vi "Write Display settings.vi"(8 "error in (no error)":errorcluster, 10 "Display settings":T1={"Min. Thresh."=0.0, "X"=0.0, "Y"=0.0, "ShowLineout"=FALSE, "ScaleParts"=10, "ShowLegende"=FALSE, "Target Cross"=FALSE, "Centroid Cross"=FALSE, "Target color"=16777226, "Centroid color"=16711680, "calibr. µm/px"=0.0}, 11 "Display Settings Dialog in":refnum<class "Display Settings Dialog.lvclass">) -> (0 "error out":errorcluster, 3 "Display Settings Dialog out":refnum<class "Display Settings Dialog.lvclass">)   [LabVIEW 2014, in "Display Settings Dialog.lvlib" / "Display Settings Dialog.lvclass"]
uses:
  Display Settings Dialog.lvclass
  HIJ Vision Display/HIJ Vision Display/DisplaySettings.ctl
  Display Settings Dialog.lvclass/Display Settings Dialog.ctl
  HIJ Vision Display/HIJ Vision Display/HIJ Vision Display.lvclass
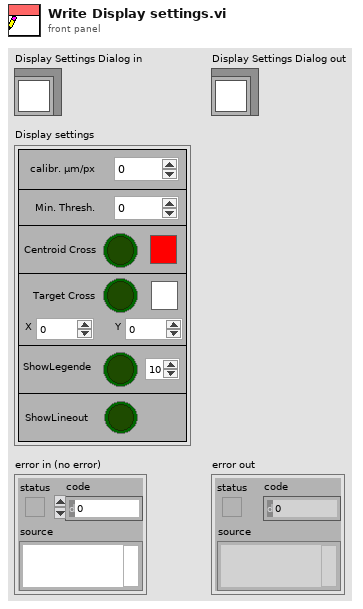
[diagram p1: front panel]
types:
  T1 = typedef "HIJ Vision Display.lvlib/HIJ Vision Display.lvclass/DisplaySettings.ctl" = cluster{"Min. Thresh.":sgl, "X":dbl, "Y":dbl, "ShowLineout":bool, "ScaleParts":i32, "ShowLegende":bool, "Target Cross":bool, "Centroid Cross":bool, "Target color":u32, "Centroid color":u32, "calibr. µm/px":sgl[unit]}
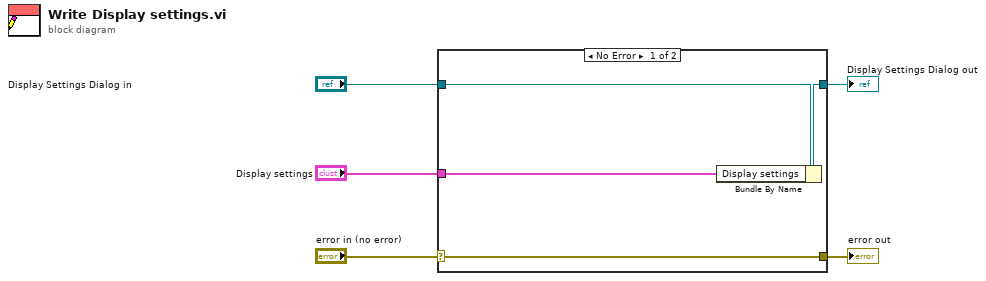
[diagram p0: block diagram]
diagram:
  n1 = case shown="No Error" "error in (no error)" {
    selector: "error in (no error)" -> [w9 w10]
    tunnel: [w9 w10] -> w4
    tunnel: [w7 w11] -> w2
    tunnel: "Display Settings Dialog in" -> [w8 w11]
    tunnel: "Display settings" -> [w6 _]
    frame No Error {
      n2 = Bundle By Name(cluster=w8, "Display settings"=w6) -> (w7:refnum<class "Display Settings Dialog.lvclass">)
    }
    frame Error {
    }
  }
  "error out" <- w4
  "Display Settings Dialog out" <- w2
